vi "Linear Average & ROI Profile.vi"() -> ()   [LabVIEW 2014]
doc: "Use this template to build a VI to use as a subVI."
uses:
  <vilib>/vision/NI_Vision_Development_Module.lvlib
panel:
  out "X Axis Averages":sgl[](graph)
  out "ROI  Profile":cluster{"x0":sgl, "dx":sgl, "Pixels Line":sgl[]}(graph)
  out "Src":T1(plugin-control)
  # ":: MVi Framework V1.0 ::\nAuthor:Gaoke Yang\nEmail: gaoke.yang@yahoo.com\nWeb: www.mvicontrol.com\nCopyright (C) 2015, MVI Technologies All Rights Reserved"
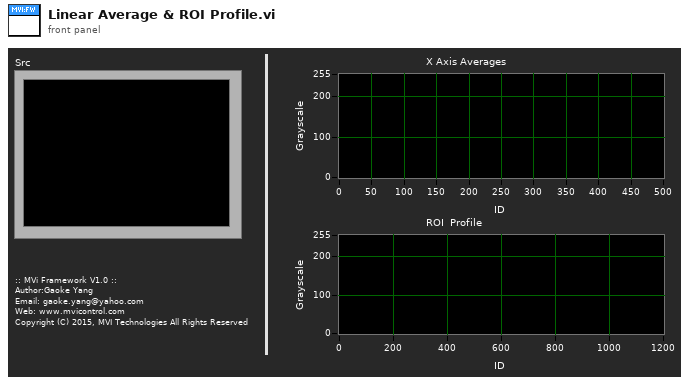
[diagram p1: front panel]
types:
  T1 = typedef "IMAQ Image.ctl" = refnum<image>
  T2 = cluster{"Global Rectangle":i32[], "Contours":cluster{"ID":enum32{"External", "Internal"}, "Type":u32, "Coordinates":i32[]}[]}
  T3 = typedef "Image Type" = u32
  T4 = typedef "IMAQ Rectangle" = cluster{"Left":i32, "Top":i32, "Right":i32, "Bottom":i32, "Rotation":dbl}
  T5 = cluster{"Left":i32, "Top":i32, "Right":i32, "Bottom":i32}
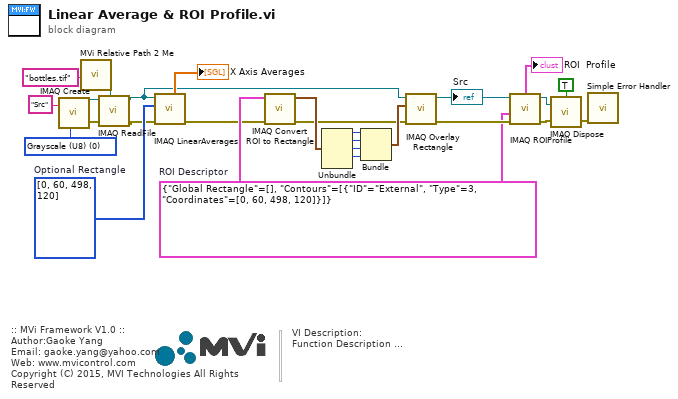
[diagram p0: block diagram]
diagram:
  w4 = i32[] [0, 60, 498, 120]  # Optional Rectangle
  w9 = T2 {"Global Rectangle"=[], "Contours"=[{"ID"=enum."External", "Type"=3, "Coordinates"=[0, 60, 498, 120]}]}  # ROI Descriptor
  w19 = T3 0 items=["Grayscale (U8)", "Grayscale (I16)", "Grayscale (SGL)", "Complex (CSG)", "RGB (U32)", "HSL (U32)", "RGB (U64)", "Grayscale (U16)"] ("Image Type")
  # "VI Description:\nFunction Description ..."
  # ":: MVi Framework V1.0 ::\nAuthor:Gaoke Yang\nEmail: gaoke.yang@yahoo.com\nWeb: www.mvicontrol.com\nCopyright (C) 2015, MVI Technologies All Rights Reserved"
  n1 = call "IMAQ Create"("Image Name"="Src" ("name or relative path"), "Image Type"=w19) -> ("New Image"=w20:T1, "error out"=w18:errorcluster)  [unwired: 2 in, 1 out]
  n2 = call "MVi Relative Path 2 Me.vi"("Relative Path"="bottles.tif" ("name or relative path")) -> ("Appended Dir"=w21:path)  [unwired: 5 in, 1 out]
  n3 = call "IMAQ ReadFile"("File Path"=w21, "error in (no error)"=w18, "Image"=w20) -> ("error out"=w2:errorcluster, "Image Out"=w3:T1)  [unwired: 4 in, 3 out]
  n4 = call "IMAQ LinearAverages"("error in (no error)"=w2, "Optional Rectangle"=w4, "Image Src"=w3) -> ("error out"=w8:errorcluster, "X Axis Averages"=→"X Axis Averages":sgl[])  [unwired: 4 in, 3 out]
  n5 = call "IMAQ Convert ROI to Rectangle"("error in (no error)"=w8, "ROI Descriptor"=w9) -> ("error out"=w6:errorcluster, "Rectangle"=w7:T4)  [unwired: 7 in]
  n6 = Unbundle(w7) -> ("Left"=w15:i32, "Top"=w14:i32, "Right"=w13:i32, "Bottom"=w12:i32)  [unwired: 1 out]
  n7 = Bundle("Left"=w15, "Top"=w14, "Right"=w13, "Bottom"=w12) -> (w11:T5)  [unwired: 1 in]
  n8 = call "IMAQ Overlay Rectangle"("error in (no error)"=w6, "Rectangle"=w11, "Image"=w3) -> ("error out"=w10:errorcluster, "Image Out"=w1:T1)  [unwired: 7 in]
  "Src" <- w1
  n9 = call "IMAQ ROIProfile"("error in (no error)"=w10, "ROI Descriptor"=w9, "Image"=w1) -> ("error out"=w17:errorcluster, "ROI Graph"=→"ROI  Profile":cluster{"x0":sgl, "dx":sgl, "Pixels Line":sgl[]})  [unwired: 1 in, 3 out]
  n10 = call "IMAQ Dispose"("All Images? (No)"=TRUE, "Image"=w1, "error in (no error)"=w17) -> ("error out"=w22:errorcluster)  [unwired: 3 out]
  n11 = call <vilib>:"Simple Error Handler.vi"("error in (no error)"=w22) -> ()  [unwired: 1 in, 8 out]
